vi "Scratch - Texture Mapping Test 1.vi"() -> ()   [LabVIEW 2022 SP3, in "3D.lvlib"]
uses:
  3D.lvlib
  Utility/Utility.lvlib
  Raster/Raster.lvlib
  Vector 3D.ctl
  Triangle 3D With Colour.ctl
  Raster/Rectangle Dimensions.ctl
  Camera.ctl
panel:
  in  "x Rotation":sgl(slide) scale=-180.0..180.0
  in  "y Rotation":sgl(slide) scale=-180.0..180.0
  in  "z Rotation":sgl(slide) scale=-180.0..180.0
  in  "x Transform":sgl(slide) scale=-10.0..10.0
  in  "y Transform":sgl(slide)=5.0 scale=-10.0..10.0
  in  "z Transform":sgl(slide)=-10.0 scale=-10.0..10.0
  out "2D Picture 2":picture
  out "2D Picture":picture
  in  "Path":path
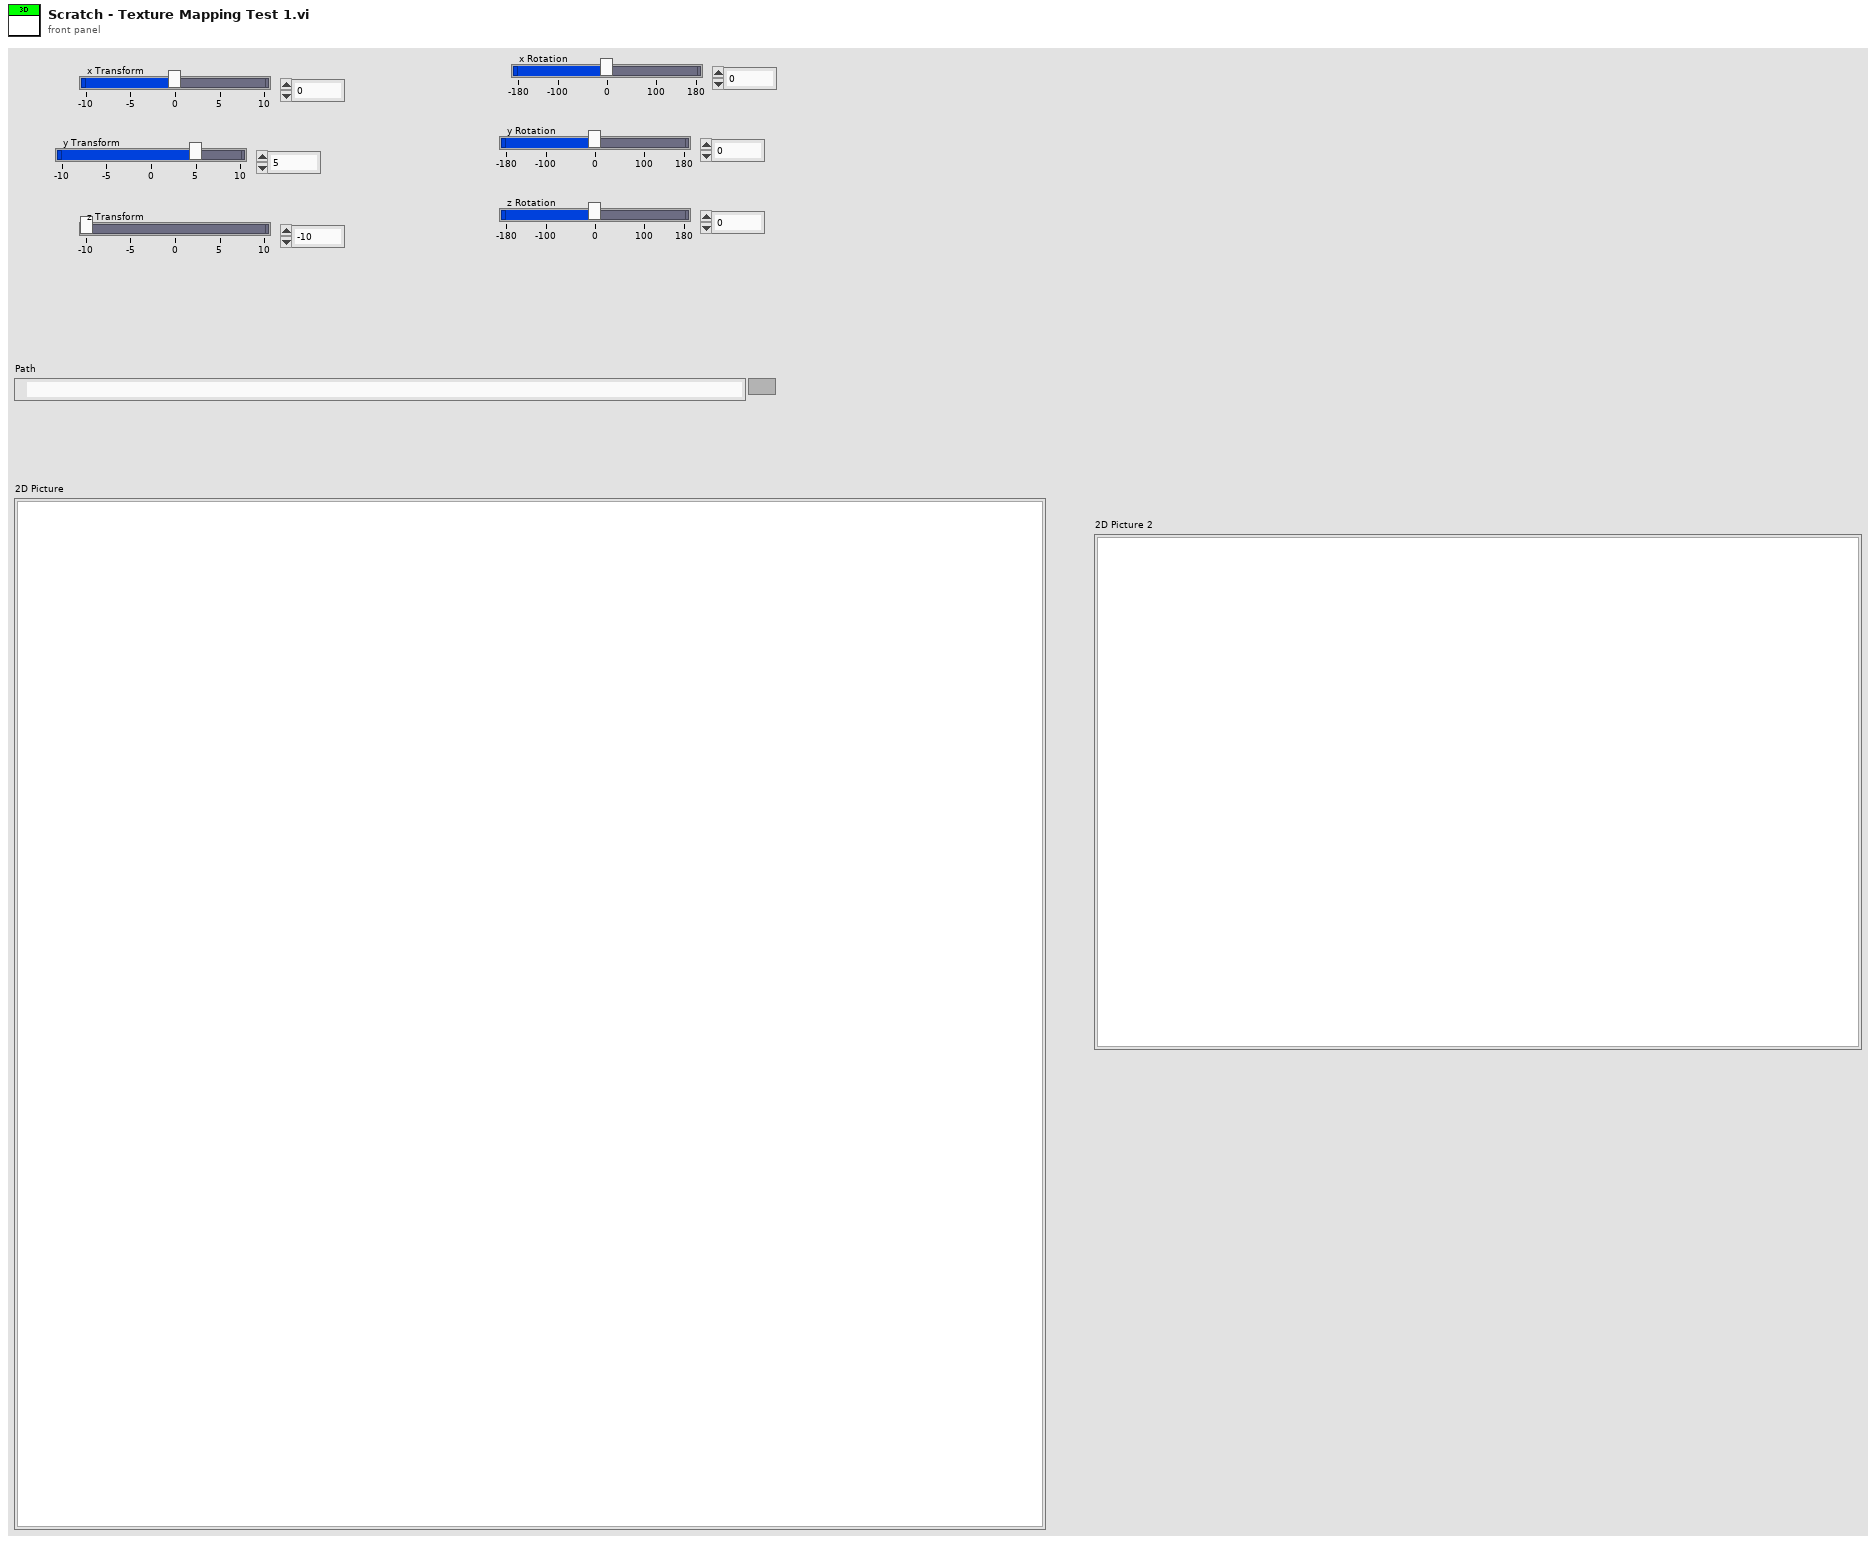
[diagram p1: front panel]
types:
  T1 = typedef "3D.lvlib/Vector 3D.ctl" = cluster{"x":sgl, "y":sgl, "z":sgl}
  T2 = typedef "3D.lvlib/Camera.ctl" = cluster{"Field Of View":sgl, "Near Plane":sgl, "Far Plane":sgl}
  T3 = typedef "Raster.lvlib/Rectangle Dimensions.ctl" = cluster{"Width":u32, "Height":u32}
  T4 = typedef "3D.lvlib/Object.ctl" = cluster{"Triangles":T5[], "Diffuse Colour":u32, "Transform":T6, "Name":string, "Alpha Blending Enabled":bool, "Alpha":dbl, "Turntable Enabled":bool, "Textures":T5[]}
  T5 = typedef "3D.lvlib/Triangle 3D.ctl" = cluster{"Point 1":T1, "Point 2":T1, "Point 3":T1}
  T6 = typedef "3D.lvlib/Transform.ctl" = cluster{"Position":T1, "Rotation":T1, "Scale":T1}
  T7 = typedef "3D.lvlib/Triangle 3D With Colour.ctl" = cluster{"Point 1":T1, "Point 2":T1, "Point 3":T1, "Fill Colour":u32, "Alpha":dbl, "Alpha Blending Enabled":bool, "Index":i32}
  T8 = typedef "3D.lvlib/Triangle 2D.ctl" = cluster{"Point 1":T9, "Point 2":T9, "Point 3":T9, "Fill Colour":u32, "Alpha":dbl, "Alpha Blending Enabled":bool, "Texture 1":T9, "Texture 2":T9, "Texture 3":T9}
  T9 = typedef "3D.lvlib/Point 2D.ctl" = cluster{"x":sgl, "y":sgl}
  T10 = typedef "imagedata.ctl" = cluster{"image type":i32, "image depth":i32, "image":u8[], "mask":u8[], "colors":u32[], "Rectangle":cluster{"left":i16, "top":i16, "right":i16, "bottom":i16}}
  T11 = typedef "Raster.lvlib/Point 2D.ctl" = cluster{"x":i32, "y":i32}
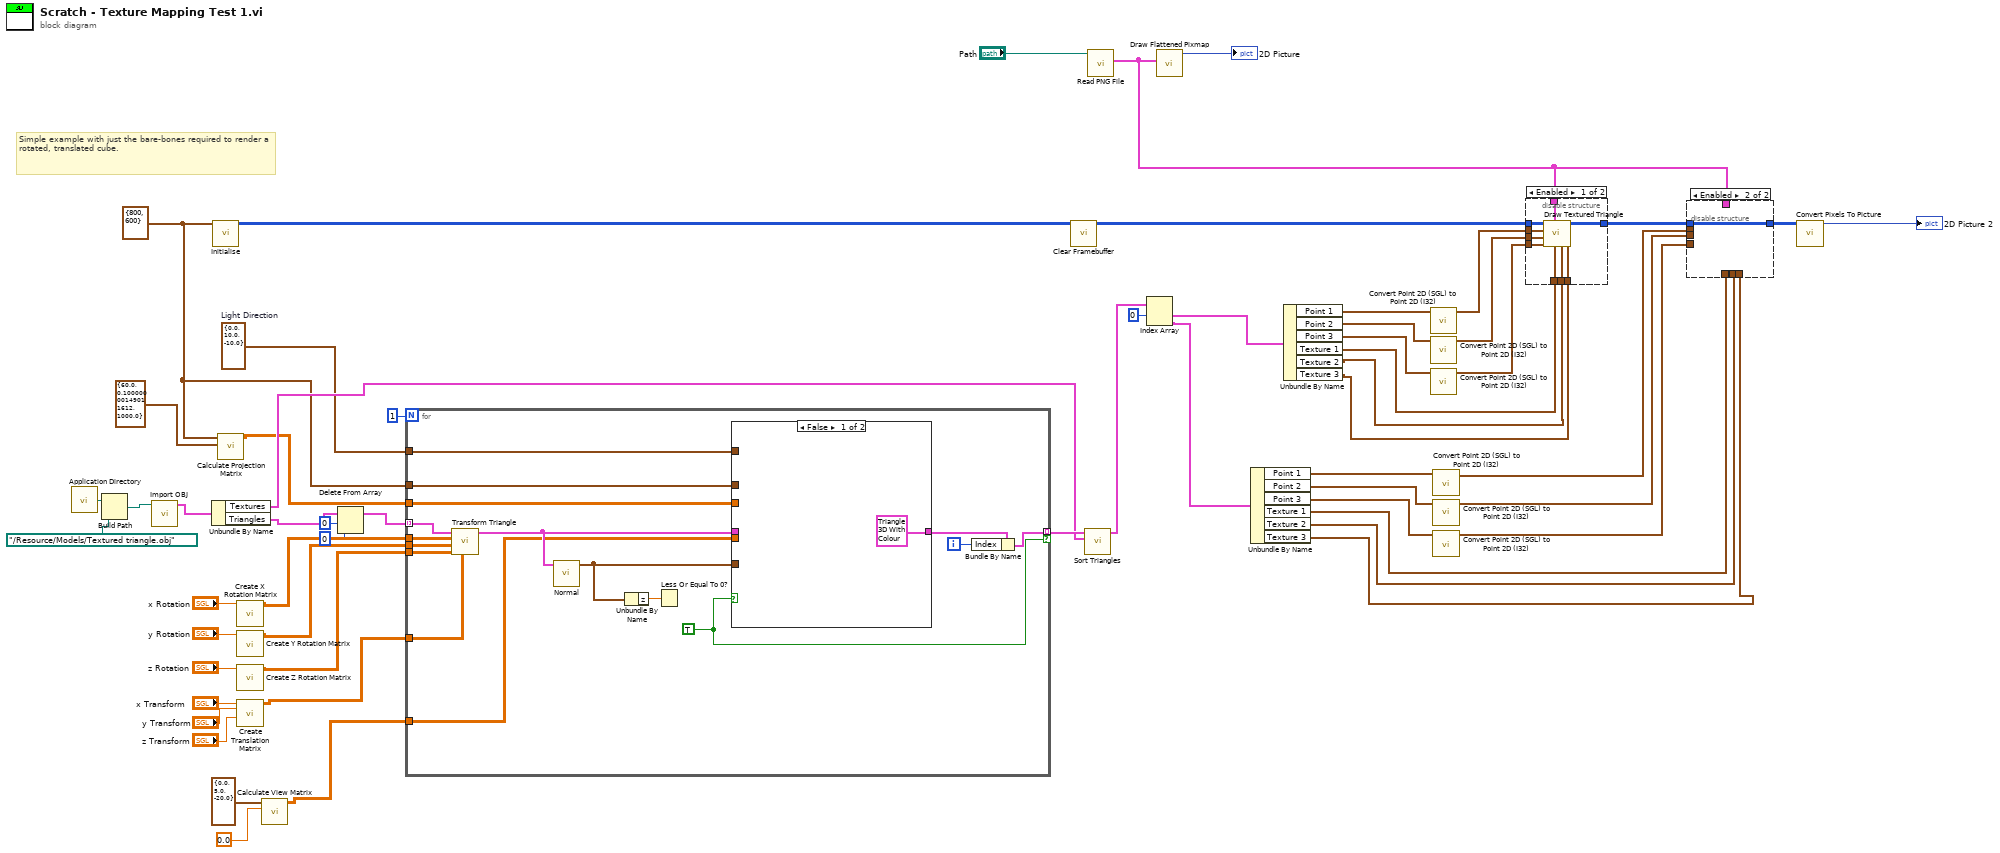
[diagram p0: block diagram]
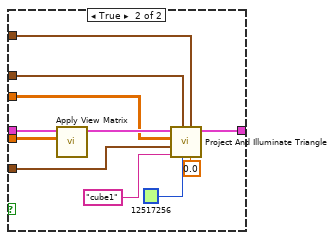
[diagram p2: hidden frame]
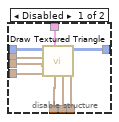
[diagram p3: hidden frame]
diagram:
  w8 = T1 {"x"=0.0, "y"=10.0, "z"=-10.0}  # Light Direction
  w9 = T3 {"Width"=800, "Height"=600} ("Screen Dimensions")
  # "Simple example with just the bare-bones required to render a rotated, translated cube."
  n1 = call <vilib>:"Application Directory.vi"() -> ("Application Directory"=w29:path)
  n2 = Build Path(base path=w29, name or relative path=path "../Resource/Models/Textured triangle.obj") -> (appended path=w30:path)
  n3 = call "Import OBJ.vi"("Object"=w30) -> ("Object"=w22:T4)  [unwired: 9 in, 1 out]
  n4 = Unbundle By Name(w22) -> ("Textures"=w11:T5[], "Triangles"=w4:T5[])
  n5 = call "Initialise.vi"("Screen Dimensions"=w9) -> ("Pixel Data out"=w13:u32[][])  [unwired: 10 in]
  n6 = call "Calculate Projection Matrix.vi"("Camera"=T2 {"Field Of View"=60.0, "Near Plane"=0.1, "Far Plane"=1000.0}, "Screen Dimensions"=w9) -> ("Projection Matrix"=w7:sgl[][])  [unwired: 9 in]
  n7 = call "Create X Rotation Matrix.vi"("Theta (°)"="x Rotation") -> ("Rotation X Matrix"=w21:sgl[][])  [unwired: 10 in]
  n8 = call "Create Y Rotation Matrix.vi"("Theta (°)"="y Rotation") -> ("Rotation Y Matrix"=w20:sgl[][])  [unwired: 10 in]
  n9 = call "Create Z Rotation Matrix.vi"("Theta (°)"="z Rotation") -> ("Rotation Z Matrix"=w19:sgl[][])  [unwired: 10 in]
  n10 = call "Create Translation Matrix.vi"("z"="z Transform", "y"="y Transform", "x"="x Transform") -> ("Translation Matrix"=w18:sgl[][])  [unwired: 8 in]
  n11 = call "Calculate View Matrix.vi"("Camera Rotation"=sgl 0.0, "Camera Position"=T1 {"x"=0.0, "y"=5.0, "z"=-20.0} ("output cluster")) -> ("View Matrix"=w15:sgl[][])  [unwired: 9 in]
  n12 = Delete From Array(array=w4, length=0, index=0) -> (array with subset deleted=w3:T5[])  [unwired: 1 out]
  n13 = for {
    N: 1 -> [_]
    tunnel: w19 -> [w71]
    tunnel: w21 -> [w73]
    tunnel: [w61] -> w12 mode=indexing if=w59
    tunnel: w20 -> [w72]
    tunnel: w18 -> [w70]
    tunnel: w3 -> [w63] mode=indexing
    tunnel: w9 -> [w68]
    tunnel: w7 -> [w67]
    tunnel: w8 -> [w66]
    tunnel: w15 -> [w64]
    i -> [w60]
    w59 = TRUE
    n14 = call "Transform Triangle.vi"("Translation Matrix"=w70, "Rotation Z Matrix"=w71, "Rotation Y Matrix"=w72, "Rotation X Matrix"=w73, "Triangle in"=w63) -> ("Triangle out"=w69:T5)  [unwired: 6 in]
    n15 = call "Normal.vi"("Triangle"=w69) -> ("Normal"=w74:T1)  [unwired: 10 in]
    n16 = Unbundle By Name(w74) -> ("z"=w65:sgl)
    n17 = Less Or Equal To 0?(x=w65) -> ()  [unwired: 1 out]
    n18 = case shown="False" w59 {
      tunnel: [T7 {"Point 1"={"x"=0.0, "y"=0.0, "z"=0.0}, "Point 2"={"x"=0.0, "y"=0.0, "z"=0.0}, "Point 3"={"x"=0.0, "y"=0.0, "z"=0.0}, "Fill Colour"=12517256, "Alpha"=0.0, "Alpha Blending Enabled"=FALSE, "Index"=0} ("Triangle") w80] -> w62
      tunnel: w74 -> [_ w86]
      tunnel: w69 -> [_ w84]
      tunnel: w68 -> [_ w83]
      tunnel: w67 -> [_ w82]
      tunnel: w66 -> [_ w81]
      tunnel: w64 -> [_ w79]
      frame False {
      }
      frame True {
        n19 = call "Apply View Matrix.vi"("View Matrix"=w79, "Triangle in"=w84) -> ("Triangle"=w85:T5)  [unwired: 9 in]
        n20 = call "Project And Illuminate Triangle.vi"("Alpha"=0.0, "Light Direction"=w81, "Diffuse Colour"=u32 12517256, "Screen Dimensions"=w83, "Name"="cube1", "Normal"=w86, "Projection Matrix"=w82, "Triangle in"=w85) -> ("Triangle"=w80:T7)  [unwired: 3 in]
      }
    }
    n21 = Bundle By Name(cluster=w62, "Index"=w60) -> (w61:T7)
  }
  n22 = call "Clear Framebuffer.vi"("Pixel Data in"=w13) -> ("Pixel Data out"=w55:u32[][])  [unwired: 10 in]
  n23 = call "Sort Triangles.vi"("Textures"=w11, "Triangles"=w12) -> ("Triangles Sorted"=w10:T8[])  [unwired: 9 in]
  n24 = call <vilib>:"Read PNG File.vi"("path to PNG file"="Path") -> ("image data"=w47:T10)  [unwired: 8 in, 2 out]
  n25 = Index Array(array=w10, index #1=0 ("index")) -> (element #1=w51:T8, element #2=w40:T8)  [unwired: 1 in]
  n26 = call <vilib>:"Draw Flattened Pixmap.vi"("image data"=w47) -> ("new picture"=→"2D Picture":picture)  [unwired: 8 in]
  n27 = Unbundle By Name(w40) -> ("Point 1"=w39:T9, "Point 2"=w38:T9, "Point 3"=w37:T9, "Texture 1"=w33:T9, "Texture 2"=w32:T9, "Texture 3"=w31:T9)
  n28 = Unbundle By Name(w51) -> ("Point 1"=w54:T9, "Point 2"=w53:T9, "Point 3"=w52:T9, "Texture 1"=w43:T9, "Texture 2"=w42:T9, "Texture 3"=w41:T9)
  n29 = call "Convert Point 2D (SGL) to Point 2D (I32).vi"("Point 2D (Float)"=w54) -> ("Point 2D (I32)"=w46:T11)  [unwired: 10 in]
  n30 = call "Convert Point 2D (SGL) to Point 2D (I32).vi"("Point 2D (Float)"=w53) -> ("Point 2D (I32)"=w45:T11)  [unwired: 10 in]
  n31 = call "Convert Point 2D (SGL) to Point 2D (I32).vi"("Point 2D (Float)"=w52) -> ("Point 2D (I32)"=w44:T11)  [unwired: 10 in]
  n32 = call "Convert Point 2D (SGL) to Point 2D (I32).vi"("Point 2D (Float)"=w39) -> ("Point 2D (I32)"=w36:T11)  [unwired: 10 in]
  n33 = call "Convert Point 2D (SGL) to Point 2D (I32).vi"("Point 2D (Float)"=w38) -> ("Point 2D (I32)"=w35:T11)  [unwired: 10 in]
  n34 = call "Convert Point 2D (SGL) to Point 2D (I32).vi"("Point 2D (Float)"=w37) -> ("Point 2D (I32)"=w34:T11)  [unwired: 10 in]
  n35 = disable-structure shown="Enabled" {
    disable-tunnel: w55 -> [w95 w96]
    disable-tunnel: w46 -> [w94 _]
    disable-tunnel: w45 -> [w93 _]
    disable-tunnel: w44 -> [w92 _]
    disable-tunnel: [w91 w96] -> w49
    disable-tunnel: w43 -> [w90 _]
    disable-tunnel: w42 -> [w89 _]
    disable-tunnel: w41 -> [w88 _]
    disable-tunnel: w47 -> [w87 _]
    frame Enabled {
      n36 = call "Draw Textured Triangle.vi"("Texture 3"=w88, "Texture 2"=w89, "Texture 1"=w90, "Texture"=w87, "Point 3"=w92, "Point 2"=w93, "Point 1"=w94, "Pixel Data in"=w95) -> ("Pixel Data out"=w91:u32[][])  [unwired: 3 in]
    }
    frame Disabled {
    }
  }
  n37 = disable-structure shown="Enabled" {
    disable-tunnel: w49 -> [w105 w106]
    disable-tunnel: [w104 w106] -> w48
    disable-tunnel: w47 -> [w103 _]
    disable-tunnel: w36 -> [w102 _]
    disable-tunnel: w35 -> [w101 _]
    disable-tunnel: w34 -> [w100 _]
    disable-tunnel: w33 -> [w99 _]
    disable-tunnel: w32 -> [w98 _]
    disable-tunnel: w31 -> [w97 _]
    frame Disabled {
      n38 = call "Draw Textured Triangle.vi"("Texture 3"=w97, "Texture 2"=w98, "Texture 1"=w99, "Texture"=w103, "Point 3"=w100, "Point 2"=w101, "Point 1"=w102, "Pixel Data in"=w105) -> ("Pixel Data out"=w104:u32[][])  [unwired: 3 in]
    }
    frame Enabled {
    }
  }
  n39 = call "Convert Pixels To Picture.vi"("Pixel Data in"=w48) -> ("2D Picture"=→"2D Picture 2":picture)  [unwired: 9 in, 1 out]
